vi "updateTimestamps.vi"(8 "error in (no error)":errorcluster, 11 "ILCCommunications in":refnum<class "ILCCommunications.lvclass">) -> (0 "error out":errorcluster, 3 "ILCCommunications out":refnum<class "ILCCommunications.lvclass">)   [LabVIEW 2016, in "ILCCommunications.lvclass"]
uses:
  ILCCommunications.lvclass
  ILCCommunications.lvclass/ILCCommunications.ctl
  Resources/FPGA/FPGA.lvclass
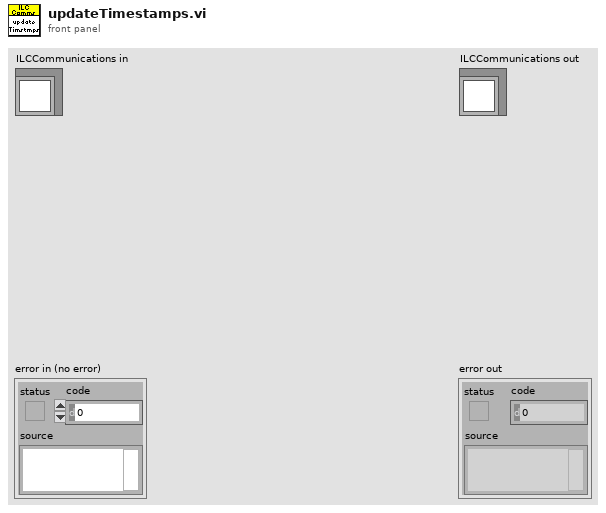
[diagram p1: front panel]
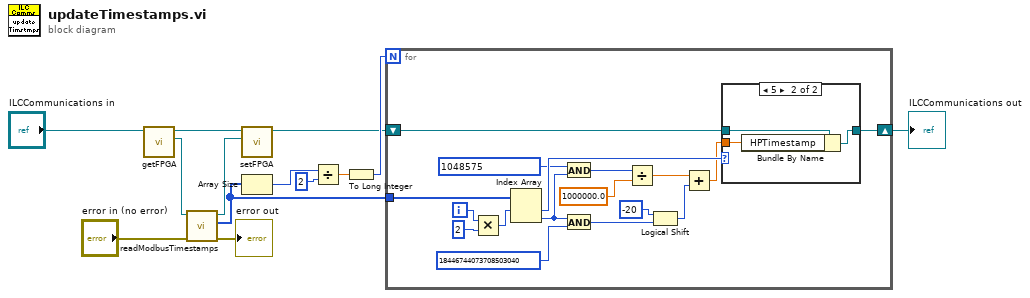
[diagram p0: block diagram]
diagram:
  n1 = call "getFPGA.vi"("ILCCommunications in"="ILCCommunications in") -> ("FPGA"=w12:refnum<class "FPGA.lvclass">, "ILCCommunications out"=w10:refnum<class "ILCCommunications.lvclass">)  [unwired: 9 in]
  n2 = call "readModbusTimestamps.vi"("error in (no error)"="error in (no error)", "FPGA in"=w12) -> ("error out"=→"error out":errorcluster, "Timestamps"=w5:u64[], "FPGA out"=w11:refnum<class "FPGA.lvclass">)  [unwired: 7 in]
  n3 = call "setFPGA.vi"("FPGA"=w11, "ILCCommunications in"=w10) -> ("ILCCommunications out"=w4:refnum<class "ILCCommunications.lvclass">)  [unwired: 9 in]
  n4 = Array Size(array=w5) -> (size(s)=w9:i32)
  n5 = Divide(x=w9, y=2) -> (x/y=w7:dbl)
  n6 = To Long Integer(number=w7) -> (32bit integer=w6:i32)
  n7 = for {
    N: w6 -> [_]
    tunnel: w5 -> [w27]
    shift-right: [w24] -> w1
    shift-left: w4 -> [w25]
    i -> [w30]
    n8 = Multiply(x=w30, y=2) -> (x*y=w28:i32)
    n9 = Index Array(array=w27, index #1=w28) -> (element #1=w26:u64, element #2=w23:u64)  [unwired: 1 in]
    n10 = And(x=u64 1048575 ("y"), y=w23) -> (x .and. y?=w17:u64)
    n11 = And(x=w23, y=u64 18446744073708503040) -> (x .and. y?=w20:u64)
    n12 = Divide(x=w17, y=1000000.0) -> (x/y=w16:dbl)
    n13 = Logical Shift(y=i16 -20, x=w20) -> (x << y=w15:u64)
    n14 = Add(x=w16, y=w15) -> (x+y=w14:dbl)
    n15 = case shown="5" w26 {
      tunnel: w14 -> [_ w33]
      tunnel: w25 -> [w31 w34]
      tunnel: [w31 w32] -> w24
      frame 0, Default {
      }
      frame 5 {
        n16 = Bundle By Name(cluster=w34, "HPTimestamp"=w33) -> (w32:refnum<class "ILCCommunications.lvclass">)
      }
    }
  }
  "ILCCommunications out" <- w1
